vi "Delay.vi"(7 "Delay Time (0)":u32 max=5000, 8 "error in (no error)":errorcluster, 11 "VISA resource name":refnum<visa-resource-name>) -> (0 "error out":errorcluster, 3 "VISA resource name out":refnum<visa-resource-name>)   [LabVIEW 2020, in "BK Precision 5491B.lvlib"]
doc: "Sets a time delay."
uses:
  <instrlib>/BK Precision 5491B/BK Precision 5491B.lvlib
panel:
  # "ms"
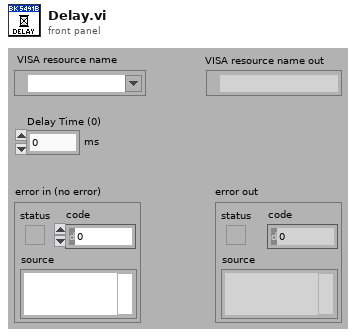
[diagram p1: front panel]
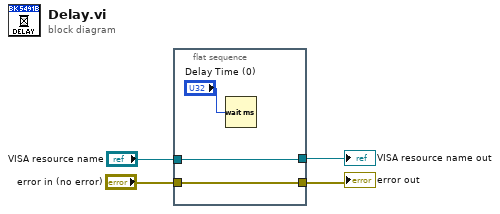
[diagram p0: block diagram]
diagram:
  n1 = flat-sequence {
    tunnel: [w6] -> w1
    tunnel: "VISA resource name" -> [w6]
    tunnel: [w5] -> w2
    tunnel: "error in (no error)" -> [w5]
    frame #0 {
      n2 = Wait (ms)(milliseconds to wait="Delay Time (0)") -> ()  [unwired: 1 out]
    }
  }
  "VISA resource name out" <- w1
  "error out" <- w2
